vi "TIFFStream Open.vi"(6 "Bytes per strip":u32=8000, 7 "File path":path, 8 "error in (no error)":errorcluster, 9 "Height Pixels":u32, 10 "Width Pixels":u32, 11 "Big endian?":bool) -> (0 "error out":errorcluster, 1 "Current and next IFD offset":u32[](array[numeric]), 2 "Image data reference":refnum<data-value>, 3 "File data":T1)   [LabVIEW 2018]
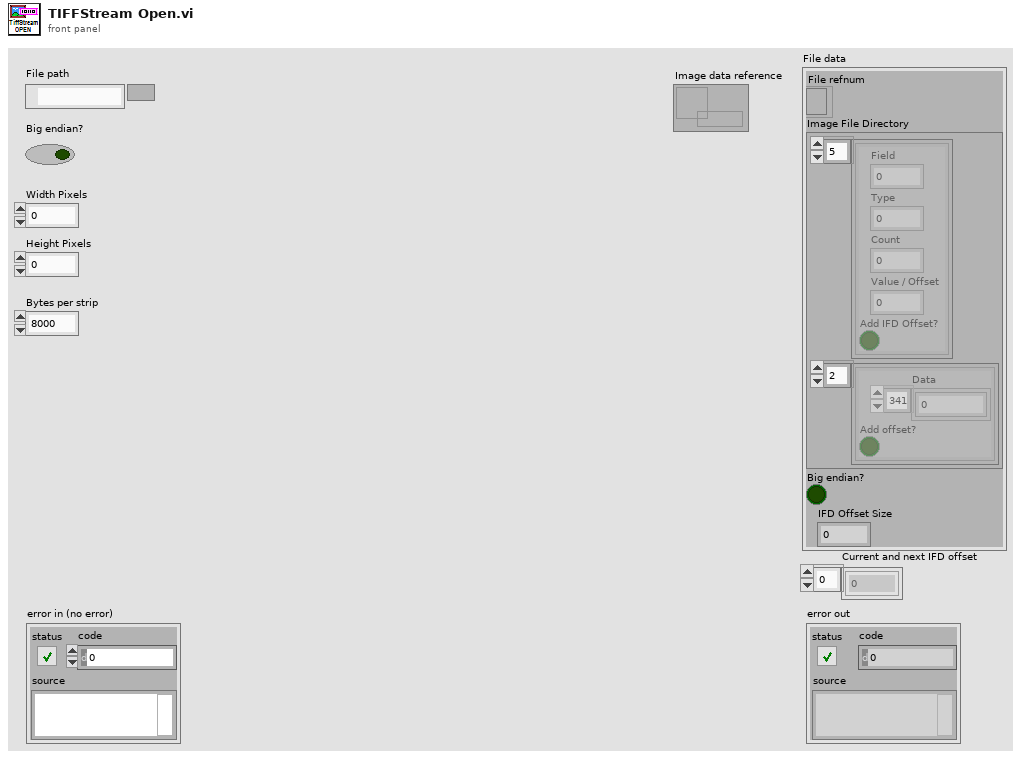
[diagram p1: front panel]
types:
  T1 = cluster{"File refnum":refnum<file>, "Image File Directory":cluster{cluster{"Field":u16, "Type":u16, "Count":u32, "Value / Offset":u32, "Add IFD Offset?":bool}[], cluster{"Data":u32[], "Add offset?":bool}[]}, "Big endian?":bool, "IFD Offset Size":u32}
  T2 = cluster{"Field":u16, "Type":u16, "Count":u32, "Value / Offset":u32, "Add IFD Offset?":bool}
  T3 = enum16{"big-endian, network order", "native, host order", "little-endian"}
  T4 = enum16{"open", "replace", "create", "open or create", "replace or create", "replace or create with confirmation"}
  T5 = cluster{"Field":u16, "Type":u16, "Count":u32, "Value / Offset":u32, "Add IFD Offset?":bool}[]
  T6 = cluster{cluster{"Field":u16, "Type":u16, "Count":u32, "Value / Offset":u32, "Add IFD Offset?":bool}[], cluster{"Data":u32[], "Add offset?":bool}[]}
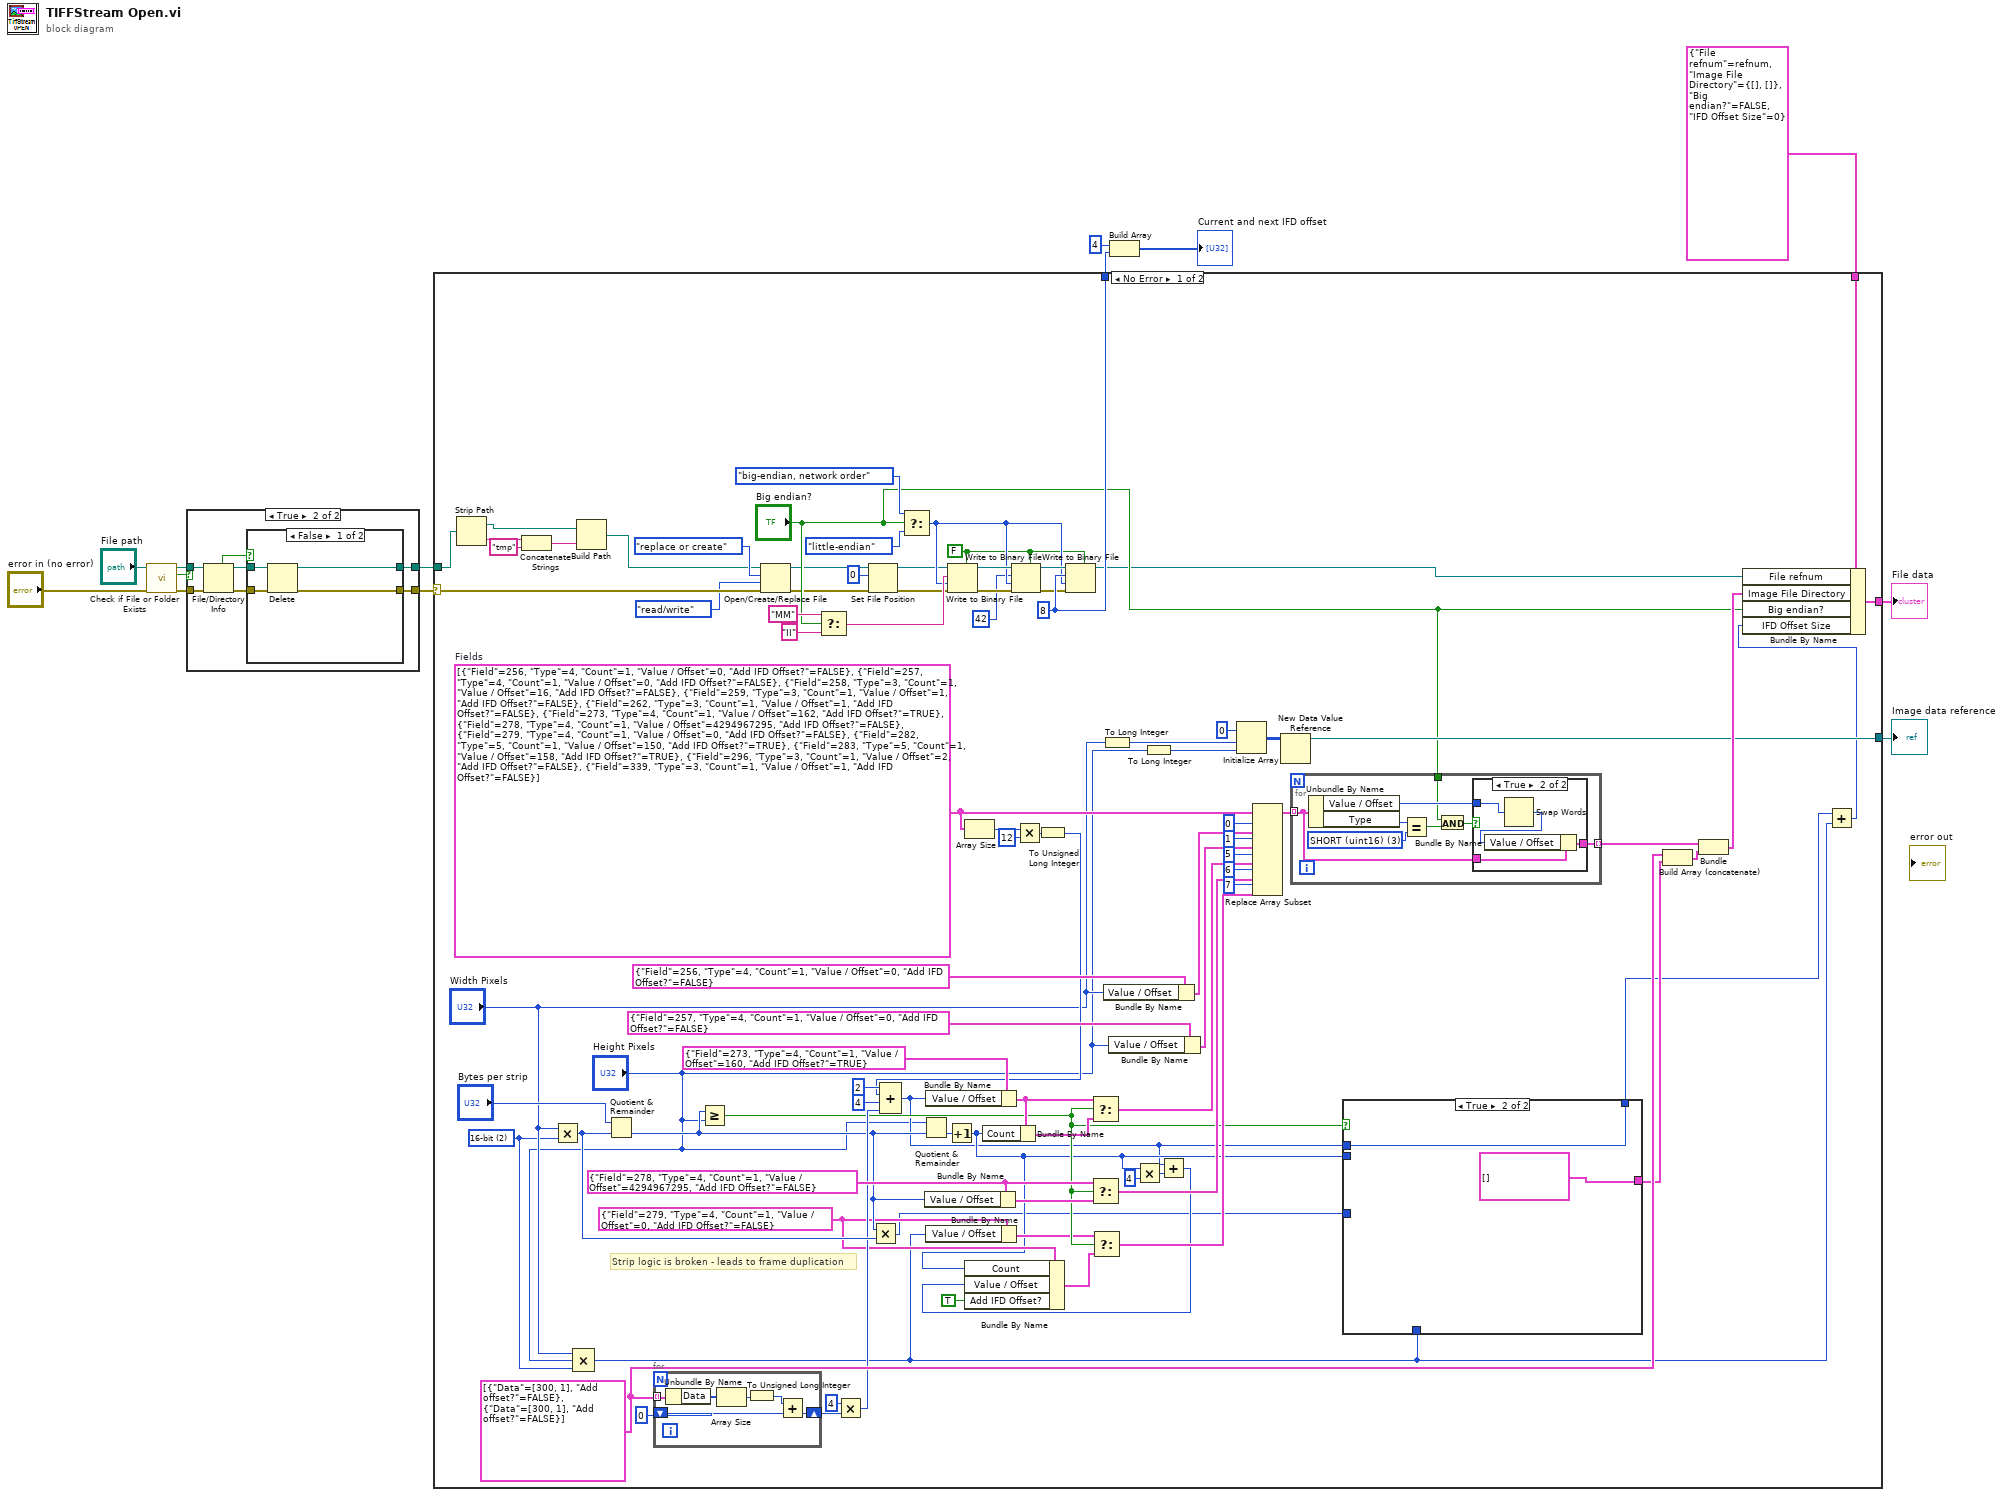
[diagram p0: block diagram]
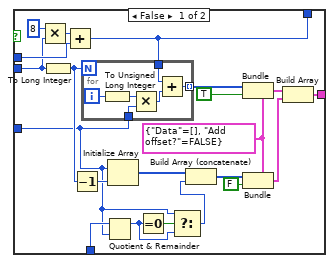
[diagram p3: hidden frame]
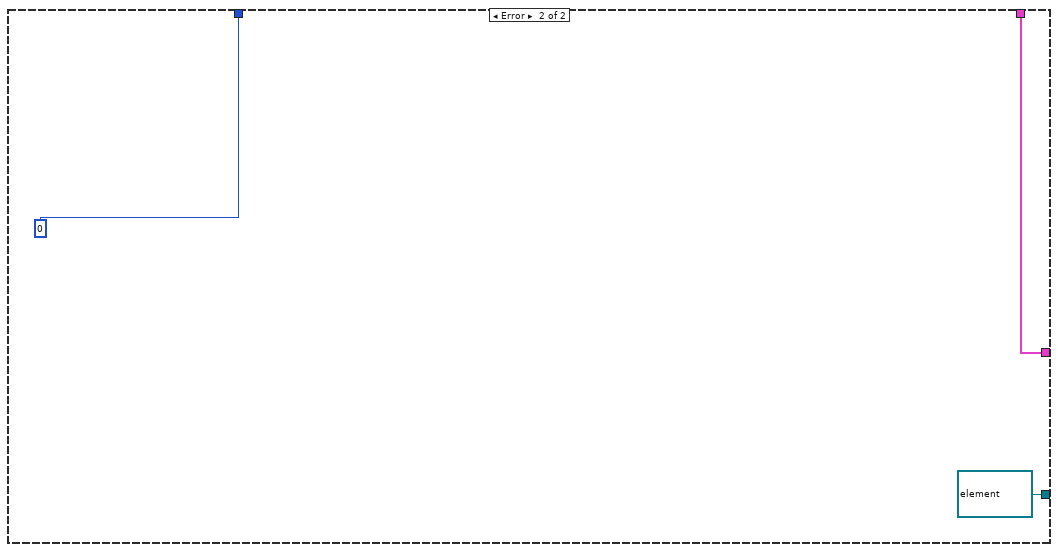
[diagram p4: hidden frame]
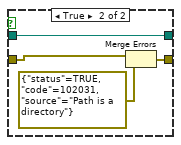
[diagram p6: hidden frame]
diagram:
  n1 = call <vilib>:"Check if File or Folder Exists.vi"("error in (no error)"="error in (no error)", "path"="File path") -> ("error out"=w11:errorcluster, "file or folder exists?"=w12:bool, "dup path"=w10:path)  [unwired: 7 in]
  n2 = case shown="True" w12 {
    tunnel: w11 -> [w15 w21]
    tunnel: w10 -> [w14 w19]
    tunnel: [w15 w22] -> w8
    tunnel: [w14 w16] -> w7
    frame False {
    }
    frame True {
      n3 = File/Directory Info(path=w19, error in=w21) -> (path out=w17:path, directory=w18:bool, error out=w20:errorcluster)  [unwired: 4 out]
      n4 = case shown="False" w18 {
        tunnel: [w26 w28] -> w22
        tunnel: w20 -> [w25 w30]
        tunnel: w17 -> [w24 w29]
        tunnel: [w23 w29] -> w16
        frame False {
          n5 = Delete(path (use dialog)=w24, error in=w25) -> (deleted path=w23:path, error out=w26:errorcluster)  [unwired: 3 in, 1 out]
        }
        frame True {
          n6 = Merge Errors(w30, errorcluster {"status"=TRUE, "code"=102031, "source"="Path is a directory"} ("error in")) -> (w28:errorcluster)
        }
      }
    }
  }
  n7 = case shown="No Error" w8 {
    selector: w8 -> [w121 _]
    tunnel: w7 -> [w38 _]
    tunnel: [w113 w172] -> w5
    tunnel: T1 {"File refnum"=refnum, "Image File Directory"={[], []}, "Big endian?"=FALSE, "IFD Offset Size"=0} ("File data") -> [w114 w172]
    tunnel: [w91 u32 0] -> w3
    tunnel: [w88 refnum<data-value> refnum ("data value reference")] -> w4
    frame No Error {
      w54 = T2 {"Field"=279, "Type"=4, "Count"=1, "Value / Offset"=0, "Add IFD Offset?"=FALSE}
      w58 = u32 2 items=["8-bit"=1, "16-bit"=2, "32-bit"=4, "64-bit"=8]
      w94 = T2 {"Field"=278, "Type"=4, "Count"=1, "Value / Offset"=4294967295, "Add IFD Offset?"=FALSE}
      w85 = cluster{"Data":u32[], "Add offset?":bool}[] [{"Data"=[300, 1], "Add offset?"=FALSE}, {"Data"=[300, 1], "Add offset?"=FALSE}]
      w86 = T5 [{"Field"=256, "Type"=4, "Count"=1, "Value / Offset"=0, "Add IFD Offset?"=FALSE}, {"Field"=257, "Type"=4, "Count"=1, "Value / Offset"=0, "Add IFD Offset?"=FALSE}, {"Field"=258, "Type"=3, "Count"=1, "Value / Offset"=16, "Add IFD Offset?"=FALSE}, {"Field"=259, "Type"=3, "Count"=1, "Value / Offset"=1, "Add IFD Offset?"=FALSE}, {"Field"=262, "Type"=3, "Count"=1, "Value / Offset"=1, "Add IFD Offset?"=FALSE}, {"Field"=273, "Type"=4, "Count"=1, "Value / Offset"=162, "Add IFD Offset?"=TRUE}, {"Field"=278, "Type"=4, "Count"=1, "Value / Offset"=4294967295, "Add IFD Offset?"=FALSE}, {"Field"=279, "Type"=4, "Count"=1, "Value / Offset"=0, "Add IFD Offset?"=FALSE}, {"Field"=282, "Type"=5, "Count"=1, "Value / Offset"=150, "Add IFD Offset?"=TRUE}, {"Field"=283, "Type"=5, "Count"=1, "Value / Offset"=158, "Add IFD Offset?"=TRUE}, {"Field"=296, "Type"=3, "Count"=1, "Value / Offset"=2, "Add IFD Offset?"=FALSE}, {"Field"=339, "Type"=3, "Count"=1, "Value / Offset"=1, "Add IFD Offset?"=FALSE}]  # Fields
      w91 = u32 8
      w70 = FALSE ("prepend array or string size? (T)")
      # "Strip logic is broken - leads to frame duplication"
      n8 = Strip Path(path=w38) -> (stripped path=w39:path, name=w42:string)
      n9 = Concatenate Strings(w42, "tmp" ("string")) -> (w40:string)
      n10 = Multiply(x="Width Pixels", y=w58) -> (x*y=w78:u32)
      n11 = Compound Arithmetic op=MULTIPLY("Width Pixels", "Height Pixels", w58) -> (w45:u32)
      n12 = Build Path(base path=w39, name or relative path=w40) -> (appended path=w32:path)
      n13 = Quotient & Remainder(x="Bytes per strip", y=w78) -> (floor(x/y)=w61:u32)  [unwired: 1 out]
      n14 = for {
        tunnel: w85 -> [w169] mode=indexing
        shift-right: [w166] -> w83
        shift-left: u32 0 -> [w165]
        n15 = Unbundle By Name(w169) -> ("Data"=w168:u32[])
        n16 = Array Size(array=w168) -> (size(s)=w167:i32)
        n17 = To Unsigned Long Integer(number=w167) -> (unsigned 32bit integer=w164:u32)
        n18 = Add(x=w164, y=w165) -> (x+y=w166:u32)
      }
      n19 = Greater Or Equal?(x=w61, y="Height Pixels") -> (x >= y?=w56:bool)
      n20 = Open/Create/Replace File(file path (use dialog)=w32, error in=w121, operation (0:open)=T4."replace or create", access (0:read/write)=enum16{"read/write", "read-only", "write-only"}."read/write") -> (refnum out=w37:refnum<file>, error out=w35:errorcluster)  [unwired: 2 in, 1 out]
      n21 = Select(t="MM", s="Big endian?", f="II") -> (s? t:f=w76:string)
      n22 = Multiply(x=u32 4, y=w83) -> (x*y=w66:u32)
      n23 = Set File Position(offset (in bytes) (0)=i64 0, refnum=w37, error in=w35) -> (refnum out=w36:refnum<file>, error out=w34:errorcluster)  [unwired: 1 in]
      n24 = Multiply(x=w61, y=w78) -> (x*y=w46:u32)
      n25 = Select(t=T3."big-endian, network order" ("byte order (0:big-endian, network order)"), s="Big endian?", f=T3."little-endian") -> (s? t:f=w71:T3)
      n26 = Quotient & Remainder(x="Height Pixels", y=w61) -> (floor(x/y)=w62:u32)  [unwired: 1 out]
      n27 = Bundle By Name(cluster=w94, "Value / Offset"=w61) -> (w93:T2)
      n28 = Bundle By Name(cluster=w54, "Value / Offset"=w45) -> (w55:T2)
      n29 = Increment(x=w62) -> (x+1=w49:u32)
      n30 = Write to Binary File(file (use dialog)=w36, data=w76, error in=w34, 5:w70, 9:w71) -> (refnum out=w73:refnum<file>, error out=w75:errorcluster)  [unwired: 1 in, 1 out]
      n31 = Array Size(array=w86) -> (size(s)=w110:i32)
      n32 = Write to Binary File(file (use dialog)=w73, data=u16 42, error in=w75, 5:w70, 9:w71) -> (refnum out=w72:refnum<file>, error out=w74:errorcluster)  [unwired: 1 in, 1 out]
      n33 = Multiply(x=w110, y=12) -> (x*y=w111:i32)
      n34 = To Unsigned Long Integer(number=w111) -> (unsigned 32bit integer=w64:u32)
      n35 = Compound Arithmetic op=ADD(u32 2 ("value"), w64, u32 4 ("value"), w66) -> (w48:u32)
      n36 = Bundle By Name(cluster=T2 {"Field"=273, "Type"=4, "Count"=1, "Value / Offset"=160, "Add IFD Offset?"=TRUE}, "Value / Offset"=w48) -> (w87:T2)
      n37 = Bundle By Name(cluster=w87, "Count"=w49) -> (w99:T2)
      n38 = Write to Binary File(file (use dialog)=w72, data=w91, error in=w74, 5:w70, 9:w71) -> (refnum out=w43:refnum<file>)  [unwired: 1 in, 2 out]
      n39 = Select(t=w87, s=w56, f=w99) -> (s? t:f=w96:T2)
      n40 = Select(t=w94, s=w56, f=w93) -> (s? t:f=w95:T2)
      n41 = To Long Integer(number="Width Pixels") -> (32bit integer=w82:i32)
      n42 = Bundle By Name(cluster=T2 {"Field"=256, "Type"=4, "Count"=1, "Value / Offset"=0, "Add IFD Offset?"=FALSE}, "Value / Offset"="Width Pixels") -> (w104:T2)
      n43 = Bundle By Name(cluster=T2 {"Field"=257, "Type"=4, "Count"=1, "Value / Offset"=0, "Add IFD Offset?"=FALSE}, "Value / Offset"="Height Pixels") -> (w103:T2)
      n44 = Multiply(x=w49, y=u32 4 ("x")) -> (x*y=w51:u32)
      n45 = To Long Integer(number="Height Pixels") -> (32bit integer=w81:i32)
      n46 = Add(x=w48, y=w51) -> (x+y=w47:u32)
      n47 = Bundle By Name(cluster=w54, "Count"=w49, "Value / Offset"=w47, "Add IFD Offset?"=TRUE) -> (w53:T2)
      n48 = Select(t=w55, s=w56, f=w53) -> (s? t:f=w57:T2)
      n49 = Initialize Array(u16 0 ("element"), w82, w81) -> (w89:u16[][])
      n50 = Replace Array Subset(array=w86, new element #1=w104, index #1=0 ("index"), new element #2=w103, index #2=1 ("index"), new element #3=w96, index #3=5 ("index"), new element #4=w95, index #4=6 ("index"), new element #5=w57, index #5=7 ("index")) -> (w68:T5)
      n51 = New Data Value Reference(data value=w89) -> (data value reference=w88:refnum<data-value>)  [unwired: 1 in, 1 out]
      n52 = for {
        tunnel: w68 -> [w126] mode=indexing
        tunnel: [w125] -> w67 mode=indexing
        tunnel: "Big endian?" -> [w122]
        w129 = u16 3 items=["BYTE (uint8)"=1, "ASCII"=2, "SHORT (uint16)"=3, "LONG (uint32)"=4, "RATIONAL (2 x LONG)"=5, "SBYTE (int8)"=6, "UNDEFINED"=7, "SSHORT (int16)"=8, "SLONG (int32)"=9, "SRATIONAL (2 x SLONG)"=10, "FLOAT"=11, "DOUBLE"=12] ("Type")
        n53 = Unbundle By Name(w126) -> ("Value / Offset"=w127:u32, "Type"=w128:u16)
        n54 = Equal?(x=w128, y=w129) -> (x = y?=w123:bool)
        n55 = And(x=w122, y=w123) -> (x .and. y?=w124:bool)
        n56 = case shown="True" w124 {
          tunnel: w127 -> [_ w132]
          tunnel: w126 -> [w130 w134]
          tunnel: [w130 w133] -> w125
          frame False {
          }
          frame True {
            n57 = Swap Words(1:w132) -> (0:w131:u32)
            n58 = Bundle By Name(cluster=w134, "Value / Offset"=w131) -> (w133:T2)
          }
        }
      }
      n59 = case shown="True" w56 {
        tunnel: w49 -> [w145 _]
        tunnel: [w152 cluster{"Data":u32[], "Add offset?":bool}[] []] -> w84
        tunnel: w46 -> [w136 _]
        tunnel: w48 -> [w149 w162]
        tunnel: [w148 w162] -> w52
        tunnel: w45 -> [w140 _]
        frame False {
          w147 = cluster{"Data":u32[], "Add offset?":bool} {"Data"=[], "Add offset?"=FALSE}
          n60 = Multiply(x=u32 8, y=w145) -> (x*y=w151:u32)
          n61 = To Long Integer(number=w145) -> (32bit integer=w144:i32)
          n62 = Add(x=w151, y=w149) -> (x+y=w148:u32)
          n63 = Decrement(x=w144) -> (x-1=w146:i32)
          n64 = for {
            N: w144 -> [_]
            tunnel: [w160] -> w155 mode=indexing
            tunnel: w148 -> [w159]
            tunnel: w136 -> [w156]
            i -> [w161]
            n65 = To Unsigned Long Integer(number=w161) -> (unsigned 32bit integer=w158:u32)
            n66 = Multiply(x=w158, y=w156) -> (x*y=w157:u32)
            n67 = Add(x=w159, y=w157) -> (x+y=w160:u32)
          }
          n68 = Quotient & Remainder(x=w140, y=w136) -> (x-y*floor(x/y)=w137:u32)  [unwired: 1 out]
          n69 = Initialize Array(w136, w146) -> (w142:u32[])
          n70 = Equal To 0?(x=w137) -> (x = 0?=w138:bool)
          n71 = Select(t=w136, s=w138, f=w137) -> (s? t:f=w135:u32)
          n72 = Build Array (concatenate)(w142, w135) -> (w141:u32[])
          n73 = Bundle(cluster=w147, "Data"=w155, "Add offset?"=TRUE) -> (w153:cluster{"Data":u32[], "Add offset?":bool})
          n74 = Bundle(cluster=w147, "Data"=w141, "Add offset?"=FALSE) -> (w139:cluster{"Data":u32[], "Add offset?":bool})
          n75 = Build Array(w153, w139) -> (w152:cluster{"Data":u32[], "Add offset?":bool}[])
        }
        frame True {
        }
      }
      n76 = Build Array (concatenate)(w85, w84) -> (w92:cluster{"Data":u32[], "Add offset?":bool}[])
      n77 = Bundle(w67, w92) -> (w112:T6)  [unwired: 1 in]
      n78 = Add(x=w52, y=w45) -> (x+y=w60:u32)
      n79 = Bundle By Name(cluster=w114, "File refnum"=w43, "Image File Directory"=w112, "Big endian?"="Big endian?", "IFD Offset Size"=w60) -> (w113:T1)
    }
    frame Error {
    }
  }
  "File data" <- w5
  "Image data reference" <- w4
  n80 = Build Array(u32 4 ("element"), w3) -> (→"Current and next IFD offset":u32[])
